vi "Read Flattener.vi"(11 "TCP Stream in":refnum<class "TCP Stream.lvclass">) -> (2 "Flattener":refnum<class "Message Flattener.lvclass">)   [LabVIEW 2020, in "TCP Stream.lvclass"]
doc: "Returns the message flattener being used when reading or writing message."
uses:
  TCP Stream.lvclass
  Abstract Classes/Message Flattener/Message Flattener.lvclass
  TCP Stream.lvclass/TCP Stream.ctl
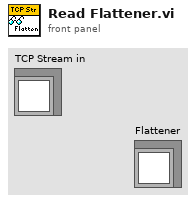
[diagram p1: front panel]
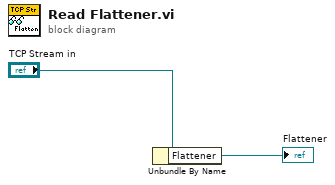
[diagram p0: block diagram]
diagram:
  n1 = Unbundle By Name("TCP Stream in") -> ("Flattener"=→"Flattener":refnum<class "Message Flattener.lvclass">)
